vi "feedback_node_basics.vi"() -> ()   [LabVIEW 2026]
panel:
  out "appended array":i16[](array[numeric])
  in  "Numeric 3":dbl
  out "Numeric 2":dbl
  in  "Numeric":dbl
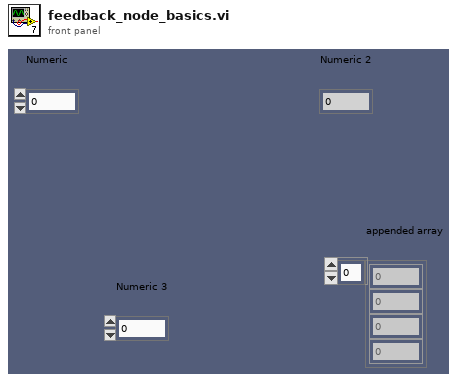
[diagram p1: front panel]
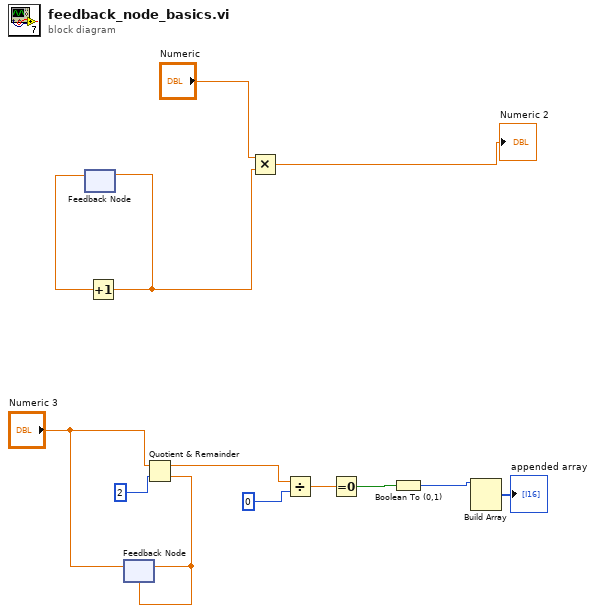
[diagram p0: block diagram]
diagram:
  n1 = feedback #1() -> (w11:dbl)  [unwired: 1 in]
  n2 = Increment(x=w11) -> (x+1=w10:dbl)
  n3 = feedback-in #1(w10) -> ()
  n4 = Quotient & Remainder(x="Numeric 3", y=2) -> (x-y*floor(x/y)=w8:dbl, floor(x/y)=w2:dbl)
  n5 = feedback-in #2(w2) -> ()
  n6 = feedback #2("Numeric 3", w2) -> ()
  n7 = Multiply(x="Numeric", y=w10) -> (x*y=→"Numeric 2":dbl)
  n8 = Divide(x=w8, y=0) -> (x/y=w6:dbl)
  n9 = Equal To 0?(x=w6) -> (x = 0?=w5:bool)
  n10 = Boolean To (0,1)(Boolean=w5) -> (0, 1=w4:i16)
  n11 = Build Array(w4) -> (→"appended array":i16[])  [unwired: 3 in]
